vi "DAQmx.vi.vi"() -> ()   [LabVIEW 2018]
uses:
  <vilib>/DAQmx/read.llb/DAQmx Read (Analog 1D Wfm NChan NSamp).vi
  <vilib>/DAQmx/configure/timing.llb/DAQmx Timing (Sample Clock).vi
  <vilib>/DAQmx/miscellaneous.llb/DAQmx Fill In Error Info.vi
panel:
  in  "Minimum time between \nreadings [ms]":u32
  in  "task/channels in":refnum<k21>="MyCurrentTask"
  out "output cluster":cluster{"data":waveform(dbl)[]}={"data"=[{"t0"=timestamp(3616718158.1640363 s since 1904-01-01), "dt"=0.001, "Y"=[-0.00018494216742454299, 0.0011462752159184545, 0.0026221503341776788, 0.0032245857112338633, 0.004788964506973479, 0.005617236854152044, 0.00739036225470748, 0.008420056764427626, 0.009322794274727621, 0.009822687459944456, 0.011247291482284006, 0.012323984496597187, 0.013559984130375072, 0.014318674275948363, 0.015240943632312997, 0.015827509384441663, 0.016251716666158024, 0.017325357829523606, 0.017139805291909543, 0.017639088106936856, 0.018515579699087497, 0.018668782616657, 0.018865321817682426, 0.01890194402905362, 0.0193511764885403, 0.019077120273445845, 0.01967955565050203, 0.01956175420392468, 0.0184850611896115, 0.018416089358195747, 0.017902157658619952, 0.01848139896847438, 0.016975005340739157, 0.016484267708365124, 0.016387218848231452, 0.016097903378399, 0.01434980315561388, 0.013934751426740319, 0.013736381115146336, 0.012425305948057496, 0.011902218695638905, 0.010953093050935392, 0.008868678853724783, 0.00880092776268807, 0.007725455488753929, 0.006078066347239601, 0.004519180883205664, 0.003783684804834132, 0.0026874599444563128, 0.001174352244636372, 9.826960051271096e-05, -0.0012048707541123692, -0.0018341624195074313, -0.0030585650196844386, -0.004505142368846705, -0.005693533127842036, -0.007275612659077731, -0.00781823175756096, -0.00977324747459334, -0.0102218695638905, -0.011466414380321664, -0.011985839411603137, -0.013660695211645863, -0.013847468489638966, -0.015246436964018678, -0.01616443372905667, -0.016937162388988923, -0.017512131107516708, -0.01813959166234321, -0.01815912350840785, -0.01878536332285531, -0.018844569231238745, -0.01867305520798364, -0.019110080263679923, -0.01944395275734733, -0.01881344035157323, -0.019343852046266062, -0.01866451002533036, -0.01909482100894192, -0.018626056703390605, -0.018226264229255044, -0.018404492324594866, -0.017794122135074922, -0.016480605487228003, -0.016028931546983247, -0.015511337626270333, -0.015251319925534837, -0.013745536667989135, -0.013393963438825648, -0.011877803888058107, -0.011657460249641408, -0.010199896237067782, -0.009250770592364269, -0.008664815210425123, -0.007148655659657582, -0.006314279610583819, -0.00499893185216834, -0.003107394634846034, -0.002324900051881466, -0.0017773979918820765], "attributes"=variant("NI_ChannelName"=variant(string "Current_0"), "NI_UnitDescription"=variant(string "Amps"))}, {"t0"=timestamp(3616718158.16405 s since 1904-01-01), "dt"=0.001, "Y"=[0.0018494216742454299, 0.0025366985076448866, 0.004047364726706748, 0.005129551072725608, 0.006358226264229255, 0.0076424451429792165, 0.009065828424939726, 0.00924100466933195, 0.010234687337870418, 0.012265999328592792, 0.012919705801568652, 0.013053376873073518, 0.014321115756706443, 0.015020599993896298, 0.016279183324686423, 0.016132694479201636, 0.01673879207739494, 0.018259834589678642, 0.017985778374584184, 0.018947111423078096, 0.018466139713736382, 0.01869197668385876, 0.019209570604571673, 0.01986083559678945, 0.018861049226355786, 0.019143650624103517, 0.018738975188451797, 0.018864711447492903, 0.0191308328501236, 0.01826349681081576, 0.017432782982879116, 0.017254554887539294, 0.01695669423505356, 0.016577043977172155, 0.015005951109347819, 0.01445600756859035, 0.013845637379070406, 0.012479628894924773, 0.012361217078157903, 0.011600085451826532, 0.010039979247413556, 0.00858851893673513, 0.007467879268776513, 0.0062343211157567064, 0.004969634083071383, 0.004422742393261513, 0.002792443617053743, 0.002183904538102359, 0.0008545182653279214, -0.0005572679830317087, -0.002132023071993164, -0.0026343577379680776, -0.0037543870357371746, -0.005565965758232368, -0.006587115085299234, -0.007257301553392132, -0.008877224036378063, -0.009960020752586445, -0.01099520859401227, -0.012368541520432142, -0.01325907162694174, -0.013957945493942076, -0.014900967436750389, -0.01583727530747398, -0.01617725150303659, -0.01620532853175451, -0.017800836207159644, -0.018309884945219276, -0.01849055452131718, -0.018983733634449294, -0.019216895046845914, -0.019648426770836513, -0.019339579454939422, -0.019479354228339487, -0.019218726157414472, -0.019413434247871335, -0.019288918729209265, -0.019485457930234686, -0.018188421277504807, -0.017791070284127325, -0.017919858394116032, -0.017550584429456464, -0.017040925321207313, -0.015768913846247748, -0.015467390972624897, -0.01477828302865688, -0.014275948362681966, -0.013352458265938292, -0.01249732963042085, -0.011471297341837824, -0.009481490524002809, -0.009436933500167851, -0.007632679219946897, -0.006617633594775231, -0.00608478041932432, -0.004511246070741905, -0.0029285561693166906, -0.0014209418012024293, -0.0001489303262428663, 0.0009826960051271096], "attributes"=variant("NI_ChannelName"=variant(string "Current_1"), "NI_UnitDescription"=variant(string "Amps"))}, {"t0"=timestamp(3616718158.164064 s since 1904-01-01), "dt"=0.001, "Y"=[0.0038331247901852473, 0.0040217291787469096, 0.005638599810785241, 0.0069234290597247235, 0.008445692312387463, 0.008783227027191993, 0.010469679860835596, 0.011375469222083193, 0.011695913571581163, 0.01337199011200293, 0.014287545396282846, 0.0143443098239082, 0.015988647114474928, 0.016754661702322458, 0.016275521103549302, 0.017206946012756737, 0.018422193060090946, 0.018422803430280466, 0.01844965971861934, 0.019595324564348277, 0.019306619464705344, 0.018994720297860652, 0.01925778984954375, 0.018878139591662343, 0.018834803308206426, 0.01857112338633381, 0.019316995757927183, 0.018187810907315288, 0.01869502853480636, 0.017637256996368297, 0.01769829401532029, 0.016597186193426313, 0.015424665059358501, 0.015704824976348154, 0.014357127597888118, 0.013830988494521928, 0.013115634632404553, 0.0113022247993408, 0.010312204351939452, 0.00912869655446028, 0.008668477431562242, 0.0069069490646076846, 0.006765953550828577, 0.005052644428846095, 0.0035798211615344707, 0.0032312997833185827, 0.0019708853419598987, 0.0006469924008911405, -0.000913113803521836, -0.002749107333597827, -0.0033539841914120914, -0.004463637195959349, -0.006142155217139195, -0.0064229255043183695, -0.007655873287148656, -0.009422894985808894, -0.009769585253456222, -0.011612292855616931, -0.012440565202795496, -0.012537614062929166, -0.01380169072542497, -0.015297708059938353, -0.01520371105075228, -0.016331064790795616, -0.016843775749992372, -0.01739188818018128, -0.01781365398113956, -0.01803460798974578, -0.018210394604327523, -0.019556260872219, -0.01914426099429304, -0.01913022247993408, -0.01948057496871853, -0.019066133610034487, -0.01955381939146092, -0.019138157292397838, -0.01869502853480636, -0.018119449446089054, -0.018001647999511705, -0.017652516251106296, -0.01760002441480758, -0.01620105594042787, -0.01621936704611347, -0.015019989623706778, -0.014338206122013001, -0.013075350199896238, -0.013119907223731193, -0.011660512100589007, -0.010386059144871364, -0.00923612170781579, -0.008662984099856563, -0.0072396008178960535, -0.006535233619190039, -0.00499893185216834, -0.0039515366069521165, -0.0032850123599963378, -0.0011139255958738975, -0.0006433301797540208, 0.0012134159367656484, 0.0027533799249244667], "attributes"=variant("NI_ChannelName"=variant(string "Current_2"), "NI_UnitDescription"=variant(string "Amps"))}, {"t0"=timestamp(3616718158.164078 s since 1904-01-01), "dt"=0.001, "Y"=[0.005484786523026215, 0.006366771446882535, 0.007199316385387738, 0.008077028717917416, 0.00924527726065859, 0.010307321390423292, 0.011377300332651753, 0.012363048188726463, 0.01315836054567095, 0.014397412030396435, 0.014985808893093661, 0.01606555375835444, 0.016139408551286354, 0.01759819330423902, 0.017775811029389323, 0.018296456801049837, 0.018976409192175053, 0.018862880336924345, 0.01856746116519669, 0.018984344004638814, 0.019213232825708793, 0.018970305490279855, 0.01891170995208594, 0.019273659474471266, 0.018784142582476272, 0.018290963469344158, 0.017896053956724754, 0.017865535447248757, 0.017996765037995546, 0.016502578814050723, 0.016105838190862757, 0.015305642872402112, 0.015057222205267494, 0.01425214392529069, 0.013110751670888394, 0.011818597979674673, 0.011139866328928496, 0.01076448866237373, 0.009315469832453384, 0.008292489394817956, 0.006598712118900113, 0.005795464949491867, 0.004944608905301065, 0.0032007812738425855, 0.002738731040375988, 0.0011279641102328562, -0.00021912289803765984, -0.0013281655323953978, -0.002881557664723655, -0.004381237220374157, -0.005150303659169286, -0.005883968626972259, -0.0071901608325449385, -0.008201544236579485, -0.009952085940122684, -0.011007415997802666, -0.011992553483687857, -0.01239051484725486, -0.013868831446272163, -0.014871059297463912, -0.015613879818109683, -0.015493636890774255, -0.016156498916592914, -0.01740653706472976, -0.018193914609210486, -0.018095645008697776, -0.01859492782372509, -0.018876918851283304, -0.01901852473525193, -0.01922116763817255, -0.018847010711996827, -0.01890621662038026, -0.019105807672353283, -0.019183324686422316, -0.018667561876277963, -0.01834162419507431, -0.018231757560960724, -0.018066957609790338, -0.0169518112735374, -0.01676686910611286, -0.016013061922055725, -0.01586901455732902, -0.015238502151554919, -0.014060487685781426, -0.013418378246406445, -0.011876583147679066, -0.01164464247566149, -0.01000274666585284, -0.008737449262977997, -0.008099612414929656, -0.007258522293771172, -0.005523850215155492, -0.004790185247352519, -0.0035370952482680746, -0.00217230750450148, -0.0007959227271340068, 0.0002142399365215003, 0.0015027314065981017, 0.0020355845820490127, 0.0038184759056367687], "attributes"=variant("NI_ChannelName"=variant(string "Current_3"), "NI_UnitDescription"=variant(string "Amps"))}, {"t0"=timestamp(3616718158.164092 s since 1904-01-01), "dt"=0.001, "Y"=[0.006969817194128239, 0.00749656666768395, 0.009015778069399091, 0.010144962920010986, 0.011048310800500503, 0.011456038087099826, 0.012640156254768517, 0.014079409161656545, 0.014213080233161413, 0.015936155278176215, 0.015626087221900082, 0.017094027527695548, 0.017676320688497574, 0.018207342753379926, 0.01836481826227607, 0.01828119754631184, 0.01920651875362407, 0.01893063142796106, 0.01902584917752617, 0.01888851588488418, 0.0189165929136021, 0.01912656025879696, 0.019420148319956053, 0.018759117404705955, 0.019187597277748956, 0.01848323007904294, 0.017789849543748282, 0.01772087771233253, 0.0163365581225013, 0.016225470748008668, 0.014959562974944303, 0.014717246009704886, 0.014038514358958708, 0.013308511612292856, 0.012219611194189276, 0.010679036835840938, 0.009289223914304026, 0.008770409253212073, 0.008171636097293008, 0.006750694296090579, 0.0049116489150669886, 0.004626606036561174, 0.002901089510788293, 0.0014551225318155461, 0.0006122013000885037, -0.0010852381969664602, -0.0024915311136204108, -0.00358592486342967, -0.0038178655354472488, -0.005519577623828853, -0.006209906308175909, -0.00739219336527604, -0.008749656666768395, -0.010082705160679953, -0.010741904965361492, -0.012009033478804896, -0.012416150395214699, -0.013743705557420575, -0.014478591265602588, -0.015142063661610767, -0.0156602679525132, -0.016992706076235237, -0.017588427381206702, -0.018245796075319683, -0.018128604998931853, -0.018452711569566942, -0.01933164464247566, -0.018848841822565385, -0.019115573595385602, -0.019728995635853144, -0.018833582567827387, -0.01953367717520676, -0.01945249794000061, -0.019309060945463422, -0.018090151676992097, -0.018754844813379315, -0.017239906002990815, -0.017111117893002105, -0.01642628254036073, -0.015915402691732534, -0.01542588579973754, -0.014073305459761345, -0.013193151646473587, -0.012671895504623554, -0.012429578539384136, -0.010386059144871364, -0.01032380138554033, -0.009296548356578265, -0.008216803491317485, -0.00597674489577929, -0.005117954039124729, -0.0044770653401287885, -0.003010345774712363, -0.0020368053224280526, -0.0008868678853724784, 0.00022339548936429945, 0.0017462691122165593, 0.0036030152287362285, 0.004164555803094577, 0.0056746116519669175], "attributes"=variant("NI_ChannelName"=variant(string "Current_4"), "NI_UnitDescription"=variant(string "Amps"))}, {"t0"=timestamp(3616718158.164106 s since 1904-01-01), "dt"=0.001, "Y"=[0.00804651020844142, 0.00977324747459334, 0.010699179052095095, 0.01151890621662038, 0.012494277779473251, 0.013277382732627338, 0.01466841639454329, 0.015074922940763572, 0.01511154515213477, 0.016144901882992033, 0.017248451185644092, 0.01695303201391644, 0.018190862758262885, 0.018933072908719137, 0.01858088930936613, 0.01903744621112705, 0.019129001739555042, 0.019620960112308114, 0.019868160039063693, 0.01956358531449324, 0.019527573473311563, 0.01914975432599872, 0.019045381023590807, 0.01901913510544145, 0.018232978301339763, 0.018094424268318737, 0.016795556505020296, 0.01600024414807581, 0.015931882686849575, 0.015293435468611713, 0.013716238898892178, 0.013404950102237006, 0.012082277901547289, 0.012018189031647693, 0.010619830927457503, 0.00978362376781518, 0.00859096041749321, 0.007293923764763329, 0.0059895626697592085, 0.004624164555803095, 0.0034424878688924833, 0.0023554185613574633, 0.001380046998504593, -0.0004119998779259621, -0.001727347636341441, -0.0025391399884029664, -0.003238013855403302, -0.004306772057252724, -0.006513260292367321, -0.0069508957182531205, -0.00858058412427137, -0.008748435926389355, -0.009868465224158452, -0.01075289162877285, -0.012009033478804896, -0.013455610827967162, -0.014685506759849849, -0.015073702200384533, -0.015928220465712455, -0.01673879207739494, -0.017224036378063294, -0.017685476241340373, -0.017446821497238075, -0.01891537217322306, -0.01858760338145085, -0.019639881588183233, -0.018870204779198582, -0.018970305490279855, -0.019845576342051453, -0.019157689138462476, -0.01944761497848445, -0.018865321817682426, -0.01879940183721427, -0.017955259865108188, -0.01836054567094943, -0.017488937040314952, -0.016796777245399335, -0.016016724143192846, -0.015764641254921108, -0.014651936399426252, -0.013994567705313272, -0.012814722128971221, -0.011866817224646747, -0.011931516464735862, -0.009856868190557573, -0.008979766228217414, -0.008850978118228705, -0.006762901699880978, -0.006505935850093082, -0.004808496353038118, -0.003652455214087344, -0.0025690481276894436, -0.0017206335642567217, -0.0004205450605792413, 0.0008203375347148045, 0.0022577593310342723, 0.0032203131199072237, 0.004834742271187475, 0.005621509445478683, 0.006921597949156163], "attributes"=variant("NI_ChannelName"=variant(string "Current_5"), "NI_UnitDescription"=variant(string "Amps"))}]}
  in  "samples per channel":i32=100
  in  "Sample Rate":dbl=1000.0 format="%0.2f"
  out "File Size":dbl=72.259765625
  out "Filepath":path=path "C:/Labview Test Data/2018-08-09/Sensors/Log_Sensors_DAQ_5.tdms"
  in  "stop":bool
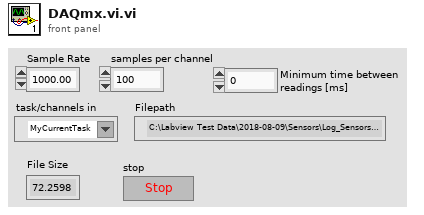
[diagram p1: front panel]
types:
  T1 = enum16{"open", "open or create", "create or replace", "create", "open (read-only)"}
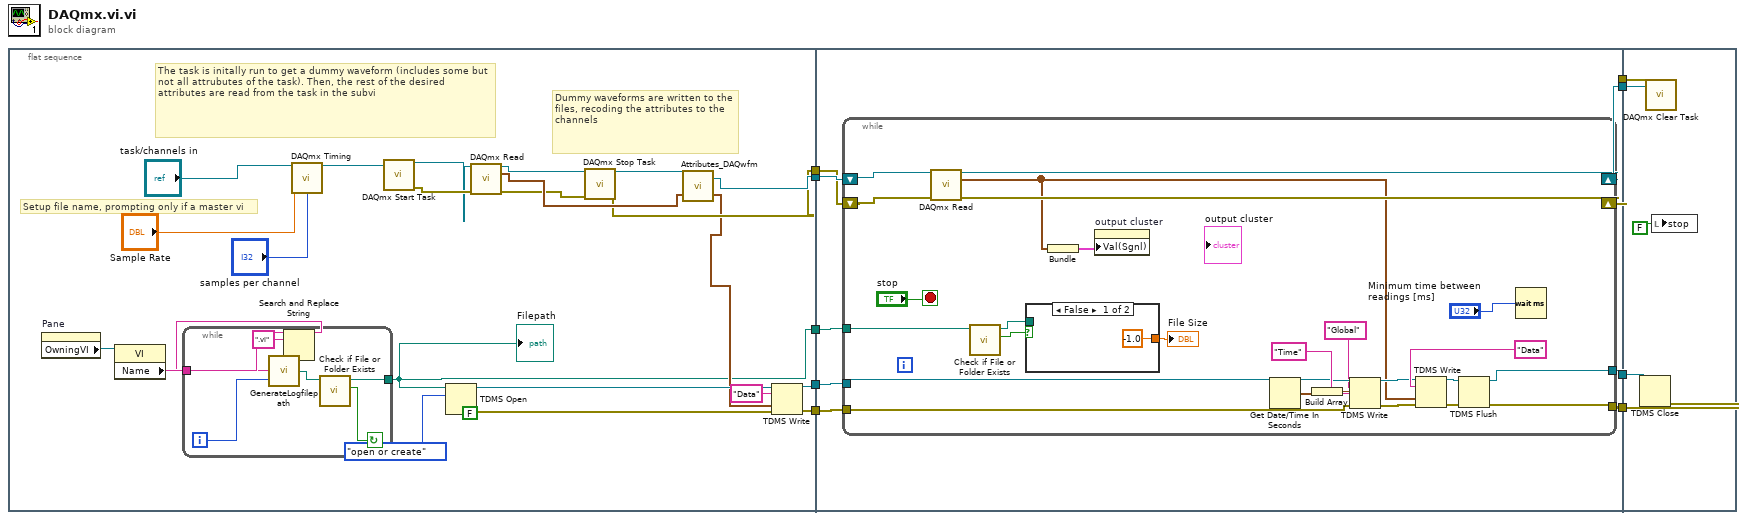
[diagram p0: block diagram]
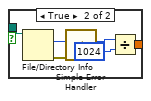
[diagram p2: hidden frame]
diagram:
  n1 = flat-sequence {
    tunnel: [w25] -> w7
    tunnel: [w24] -> w6
    tunnel: [w20] -> w5
    tunnel: [w19] -> w4
    tunnel: [w10] -> w1
    tunnel: [w48] -> w9
    tunnel: [w46] -> w8
    tunnel: w7 -> [w47]
    tunnel: w6 -> [w45]
    tunnel: w5 -> [w44]
    tunnel: w4 -> [w43]
    tunnel: [w42] -> w3
    tunnel: [w41] -> w2
    tunnel: w1 -> [w40]
    tunnel: w9 -> [w84]
    tunnel: w8 -> [w80]
    tunnel: w3 -> [w82]
    tunnel: w2 -> [w81]
    frame #0 {
      # "Setup file name, prompting only if a master vi"
      # "Dummy waveforms are written to the files, recoding the attributes to the channels"
      # "The task is initally run to get a dummy waveform (includes some but not all attrubutes of the task). Then, the rest of the desired attributes are read from the task in the subvi"
      n2 = property on="Pane" class="Pane"() -> ("OwningVI"=w34:refnum<vi>)  [unwired: 2 in, 2 out]
      n3 = property class="VI"(reference=w34) -> ("Name"=w33:string)  [unwired: 1 in, 2 out]
      n4 = Search and Replace String(input string=w33, search string=".vi") -> (result string=w14:string)  [unwired: 6 in, 3 out]
      n5 = while {
        tunnel: w14 -> [w37]
        tunnel: [w38] -> w10
        i -> [w36]
        stop <- w39 continue-if-true
        n6 = call "GenerateLogfilepath.vi"("Number"=w36, "Instrument"=w37) -> ("Logfile Path"=w35:path)
        n7 = call <vilib>:"Check if File or Folder Exists.vi"("path"=w35) -> ("file or folder exists?"=w39:bool, "dup path"=w38:path)  [unwired: 8 in, 1 out]
      }
      "Filepath" <- w10
      n8 = call-poly <vilib>:"DAQmx Timing.vi"("task/channels in"="task/channels in", "samples per channel"="samples per channel", "rate"="Sample Rate") -> ("task out"=w16:refnum<k21>)  [unwired: 11 in, 1 out]
      n9 = call <vilib>:"DAQmx Start Task.vi"("task/channels in"=w16) -> ("task out"=w27:refnum<k21>, "error out"=w28:errorcluster)  [unwired: 13 in]
      n10 = TDMS Open(5:FALSE ("create index file? (T)"), 10:T1."open or create" ("operation (0:open)"), 11:w10) -> (0:w21:errorcluster, 3:w22:refnum<k34>)  [unwired: 4 in]
      n11 = call-poly <vilib>:"DAQmx Read.vi"("task/channels in"=w27, "error in"=w28) -> ("task out"=w29:refnum<k21>, "data"=w32:waveform(dbl)[], "error out"=w30:errorcluster)  [unwired: 11 in]
      n12 = call <vilib>:"DAQmx Stop Task.vi"("task/channels in"=w29, "error in"=w30) -> ("task out"=w31:refnum<k21>, "error out"=w24:errorcluster)  [unwired: 12 in]
      n13 = call "Attributes_DAQwfm.vi"("data"=w32, "Refnum in"=w31) -> ("Array"=w12:waveform(dbl)[], "Refnum in 2"=w25:refnum<k21>)
      n14 = TDMS Write(0:w22, 5:"Data" ("group name in (Untitled)"), 9:w12, 11:w21) -> (4:w20:refnum<k34>, 15:w19:errorcluster)  [unwired: 2 in, 2 out]
    }
    frame #1 {
      n15 = while {
        shift-right: [w73] -> w48
        shift-left: w45 -> [w69]
        shift-right: [w70] -> w46
        shift-left: w47 -> [w71]
        tunnel: w44 -> [w60]
        tunnel: w43 -> [w59]
        tunnel: [w64] -> w42
        tunnel: [w63] -> w41
        tunnel: w40 -> [w49]
        stop <- "stop" stop-if-true
        n16 = call-poly <vilib>:"DAQmx Read.vi"("task/channels in"=w71, "error in"=w69) -> ("task out"=w70:refnum<k21>, "data"=w51:waveform(dbl)[], "error out"=w73:errorcluster)  [unwired: 11 in]
        n17 = call <vilib>:"Check if File or Folder Exists.vi"("path"=w49) -> ("file or folder exists?"=w56:bool, "dup path"=w57:path)  [unwired: 8 in, 1 out]
        n18 = case shown="False" w56 {
          tunnel: [-1.0 w78] -> w55
          tunnel: w57 -> [_ w75]
          frame False {
          }
          frame True {
            n19 = File/Directory Info(path=w75) -> (size=w79:i64, error out=w77:errorcluster)  [unwired: 1 in, 5 out]
            n20 = call <vilib>:"Simple Error Handler.vi"("error in (no error)"=w77) -> ()  [unwired: 1 in, 8 out]
            n21 = Divide(x=w79, y=i64 1024) -> (x/y=w78:dbl)
          }
        }
        "File Size" <- w55
        n22 = Bundle("data"=w51) -> (w50:cluster{"data":waveform(dbl)[]})  [unwired: 1 in]
        n23 = property on="output cluster" class="Clust (strict)"("Val(Sgnl)"=w50) -> ()  [unwired: 2 in, 2 out]
        n24 = Get Date/Time In Seconds() -> (seconds since 1Jan1904=w62:timestamp)
        n25 = Build Array(w62) -> (w58:timestamp[])
        n26 = TDMS Write(0:w60, 5:"Global" ("group name in (Untitled)"), 7:"Time" ("group name in (Untitled)"), 9:w58, 11:w59) -> (4:w53:refnum<k34>, 15:w52:errorcluster)  [unwired: 1 in, 2 out]
        n27 = TDMS Write(0:w53, 5:"Data" ("group name in (Untitled)"), 9:w51, 11:w52) -> (4:w66:refnum<k34>, 15:w67:errorcluster)  [unwired: 2 in, 2 out]
        n28 = TDMS Flush(4:w67, 7:w66) -> (0:w63:errorcluster, 3:w64:refnum<k34>)
        n29 = Wait (ms)(milliseconds to wait="Minimum time between \nreadings [ms]") -> ()  [unwired: 1 out]
      }
    }
    frame #2 {
      n30 = TDMS Close(8:w81, 11:w82) -> ()  [unwired: 2 out]
      n31 = call <vilib>:"DAQmx Clear Task.vi"("task in"=w80, "error in"=w84) -> ()  [unwired: 13 in, 1 out]
      n32 = local write "stop"(FALSE ("stop")) -> ()
    }
  }
